vi "H5Pset_fapl_log.vi"(5 "Buffer size":u64=1024, 6 "error in (no error)":errorcluster, 7 "Log flags":T1 items=["H5FD_LOG_NONE"=0, "H5FD_LOG_LOC_READ"=1, "H5FD_LOG_LOC_WRITE"=2, "H5FD_LOG_LOC_SEEK"=4, "H5FD_LOG_IO"=7, "H5FD_LOG_FILE_READ"=8, "H5FD_LOG_FILE_WRITE"=16, "H5FD_LOG_FILE_IO"=24, "H5FD_LOG_FLAVOR"=32, "H5FD_LOG_NUM_READ"=64, "H5FD_LOG_NUM_WRITE"=128, "H5FD_LOG_NUM_SEEK"=256, "H5FD_LOG_NUM_IO"=338, "H5FD_LOG_TIME_OPEN"=512, "H5FD_LOG_TIME_READ"=1024, "H5FD_LOG_TIME_WRITE"=2048, "H5FD_LOG_TIME_SEEK"=4096, "H5FD_LOG_TIME_CLOSE"=8192, "H5FD_LOG_TIME_IO"=15872, "H5FD_LOG_ALLOC"=16384, "H5FD_LOG_ALL"=32767], 8 "Log file":path, 9 "HDF5 Property List Ref":T2) -> (0 "error out":errorcluster, 3 "HDF5 Property List Ref out":T2)   [LabVIEW 2017]
doc: "Sets up the logging virtual file driver (H5FD_LOG) for use."
uses:
  <vilib>/UPVI/lvhdf5/library.llb/HDF5 Ref.ctl
  <vilib>/UPVI/lvhdf5/property.llb/H5FD_log_t.ctl
  <vilib>/UPVI/lvhdf5/hdf5.dll
panel:
  # "LVHDF5 Toolkit\nCopyright (c) 2005-2013 by Jason D. Sommerville\nCopyright (c) 2014 by UPVI, LLC.\n\nThis use and distribution of this file is governed by the terms found in \nLICENSE.txt distributed with this toolkit and installed at\n <user.lib>\\_lvhdf5\\LICENSE.txt"
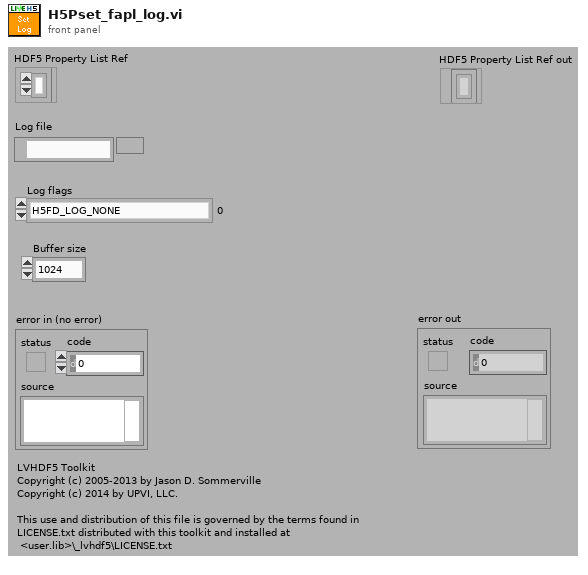
[diagram p1: front panel]
types:
  T1 = typedef "H5FD_log_t.ctl" = u64
  T2 = typedef "HDF5 Ref.ctl" = refnum<k1>
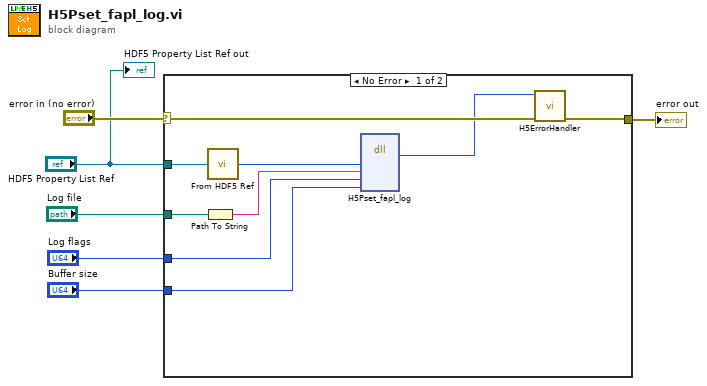
[diagram p0: block diagram]
diagram:
  n1 = case shown="No Error" "error in (no error)" {
    selector: "error in (no error)" -> [w15 w16]
    tunnel: [w14 w16] -> w5
    tunnel: "HDF5 Property List Ref" -> [w13 _]
    tunnel: "Log file" -> [w10 _]
    tunnel: "Log flags" -> [w8 _]
    tunnel: "Buffer size" -> [w7 _]
    frame No Error {
      n2 = Path To String(path=w10) -> (string=w9:string)
      n3 = call <vilib>:"From HDF5 Ref.vi"("HDF5 Ref"=w13) -> ("I32"=w12:i32)
      n4 = dll-call lib="C:/Program Files/National Instruments/LabVIEW 2017/vi.lib/UPVI/lvhdf5/hdf5.dll" fn="H5Pset_fapl_log"("plist_id"=w12, "logfile"=w9, "flags"=w8, "buf_size"=w7) -> ("return type"=w11:i32)  [unwired: 7 in, 2 out]
      n5 = call <vilib>:"H5ErrorHandler.vi"("error in (no error)"=w15, "herr_t"=w11) -> ("error out"=w14:errorcluster)  [unwired: 3 in, 4 out]
    }
    frame Error {
    }
  }
  "error out" <- w5
  "HDF5 Property List Ref out" <- "HDF5 Property List Ref"
